vi "Cfg_INTAN (SubVI).vi"(6 "INTAN 3":string, 7 "INTAN 0":string, 8 "error in (no error)":errorcluster, 9 "INTAN 2":string, 10 "INTAN 1":string, 11 "TCP Network Connection in":refnum<k5>) -> (0 "error out":errorcluster, 1 "INTAN 0 out":string, 2 "INTAN 3 out":string, 3 "TCP Network Connection out":refnum<k5>, 4 "INTAN 1 out":string, 5 "INTAN 2 out":string)   [LabVIEW 2019]
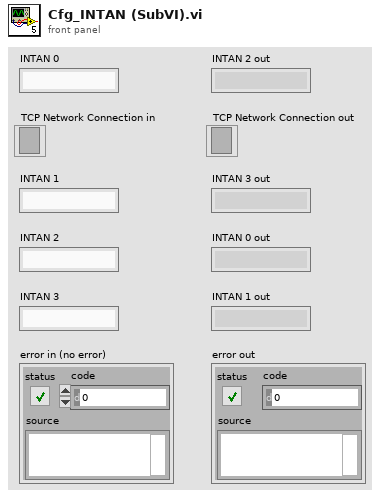
[diagram p1: front panel]
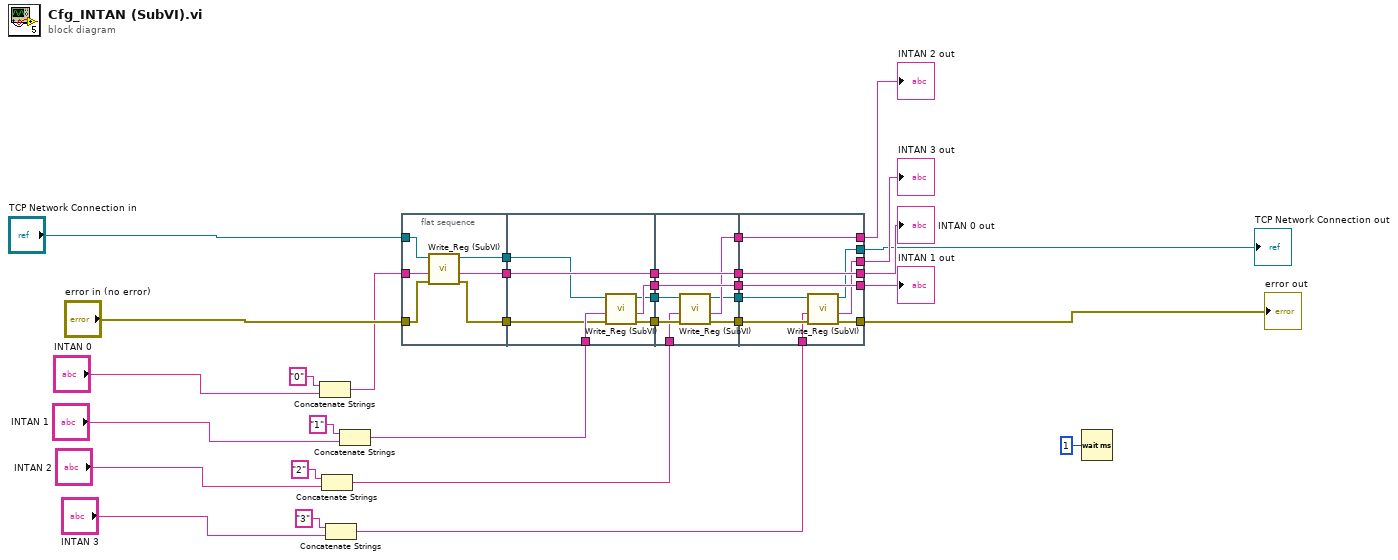
[diagram p0: block diagram]
diagram:
  n1 = Concatenate Strings("0" ("string"), "INTAN 0") -> (w12:string)
  n2 = Concatenate Strings("2" ("string"), "INTAN 2") -> (w2:string)
  n3 = Concatenate Strings("3" ("string"), "INTAN 3") -> (w6:string)
  n4 = Concatenate Strings("1" ("string"), "INTAN 1") -> (w9:string)
  n5 = flat-sequence {
    tunnel: "error in (no error)" -> [w39]
    tunnel: w12 -> [w38]
    tunnel: "TCP Network Connection in" -> [w37]
    tunnel: [w36] -> w33
    tunnel: [w35] -> w32
    tunnel: [w34] -> w31
    tunnel: w33 -> [w46]
    tunnel: w9 -> [w45]
    tunnel: [w46] -> w30
    tunnel: [w44] -> w29
    tunnel: [w43] -> w28
    tunnel: [w42] -> w27
    tunnel: w32 -> [w41]
    tunnel: w31 -> [w40]
    tunnel: w30 -> [w54]
    tunnel: w29 -> [w52]
    tunnel: w28 -> [w53]
    tunnel: w27 -> [w51]
    tunnel: [w54] -> w26
    tunnel: [w53] -> w25
    tunnel: [w50] -> w24
    tunnel: [w49] -> w23
    tunnel: [w48] -> w22
    tunnel: w2 -> [w47]
    tunnel: [w61] -> w7
    tunnel: [w62] -> w8
    tunnel: [w63] -> w10
    tunnel: w26 -> [w63]
    tunnel: w25 -> [w62]
    tunnel: w24 -> [w60]
    tunnel: w23 -> [w61]
    tunnel: w22 -> [w58]
    tunnel: w6 -> [w59]
    tunnel: [w57] -> w5
    tunnel: [w56] -> w4
    tunnel: [w55] -> w3
    frame #0 {
      n6 = call "Write_Reg (SubVI).vi"("error in (no error)"=w39, "data in"=w38, "TCP Network Connection in"=w37) -> ("error out"=w35:errorcluster, "data out"=w36:string, "TCP Network Connection out"=w34:refnum<k5>)  [unwired: 6 in]
    }
    frame #1 {
      n7 = call "Write_Reg (SubVI).vi"("error in (no error)"=w41, "data in"=w45, "TCP Network Connection in"=w40) -> ("error out"=w44:errorcluster, "data out"=w43:string, "TCP Network Connection out"=w42:refnum<k5>)  [unwired: 6 in]
    }
    frame #2 {
      n8 = call "Write_Reg (SubVI).vi"("error in (no error)"=w52, "data in"=w47, "TCP Network Connection in"=w51) -> ("error out"=w50:errorcluster, "data out"=w49:string, "TCP Network Connection out"=w48:refnum<k5>)  [unwired: 6 in]
    }
    frame #3 {
      n9 = call "Write_Reg (SubVI).vi"("error in (no error)"=w60, "data in"=w59, "TCP Network Connection in"=w58) -> ("error out"=w57:errorcluster, "data out"=w56:string, "TCP Network Connection out"=w55:refnum<k5>)  [unwired: 6 in]
    }
  }
  n10 = Wait (ms)(milliseconds to wait=u32 1) -> ()  [unwired: 1 out]
  "INTAN 0 out" <- w10
  "INTAN 1 out" <- w8
  "INTAN 2 out" <- w7
  "error out" <- w5
  "INTAN 3 out" <- w4
  "TCP Network Connection out" <- w3
